vi "Global of Tank 1.vi"() -> ()   [LabVIEW 2012]
panel:
  in  "able to shoot":bool
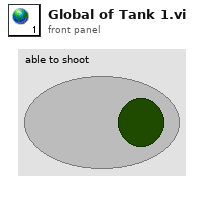
[diagram p1: front panel]
diagram:
